vi "RichToFlatlogging_service_LogRequest.vi"(5 "OutputClusterType":T1, 11 "InputCluster":T2) -> (3 "OutputCluster":T1)   [LabVIEW 2021, in "log_measurement_client.lvlib"]
uses:
  log_measurement_client.lvlib
  logging_service_LogRequest.ctl
  logging_service_LogRequest_Flat.ctl
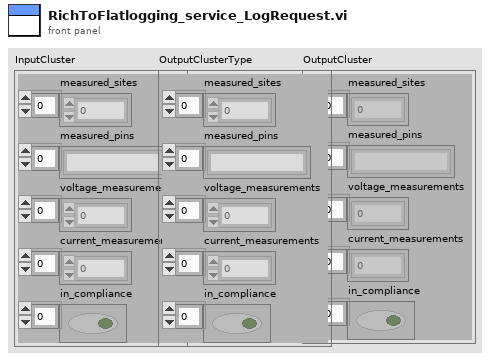
[diagram p1: front panel]
types:
  T1 = typedef "log_measurement_client.lvlib/logging_service_LogRequest_Flat.ctl" = cluster{"measured_sites":i32[], "measured_pins":string[], "voltage_measurements":sgl[], "current_measurements":sgl[], "in_compliance":bool[]}
  T2 = typedef "log_measurement_client.lvlib/logging_service_LogRequest.ctl" = cluster{"measured_sites":i32[], "measured_pins":string[], "voltage_measurements":sgl[], "current_measurements":sgl[], "in_compliance":bool[]}
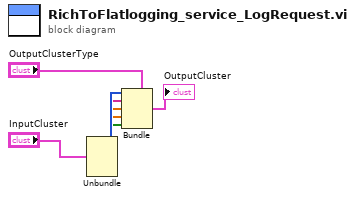
[diagram p0: block diagram]
diagram:
  n1 = Unbundle "Unbundle"("InputCluster") -> ("measured_sites"=w5:i32[], "measured_pins"=w4:string[], "voltage_measurements"=w3:sgl[], "current_measurements"=w2:sgl[], "in_compliance"=w1:bool[])
  n2 = Bundle "Bundle"(cluster="OutputClusterType", "measured_sites"=w5, "measured_pins"=w4, "voltage_measurements"=w3, "current_measurements"=w2, "in_compliance"=w1) -> (→"OutputCluster":T1)
